vi "ini_build_objects_list.vi"(8 "error in":errorcluster, 9 "VI rel path (empty)":string, 10 "VI name (empty)":string, 11 "objects":refnum<vi>[](array[refnum])) -> (0 "error out":errorcluster, 3 "objects list":string)   [LabVIEW 2013]
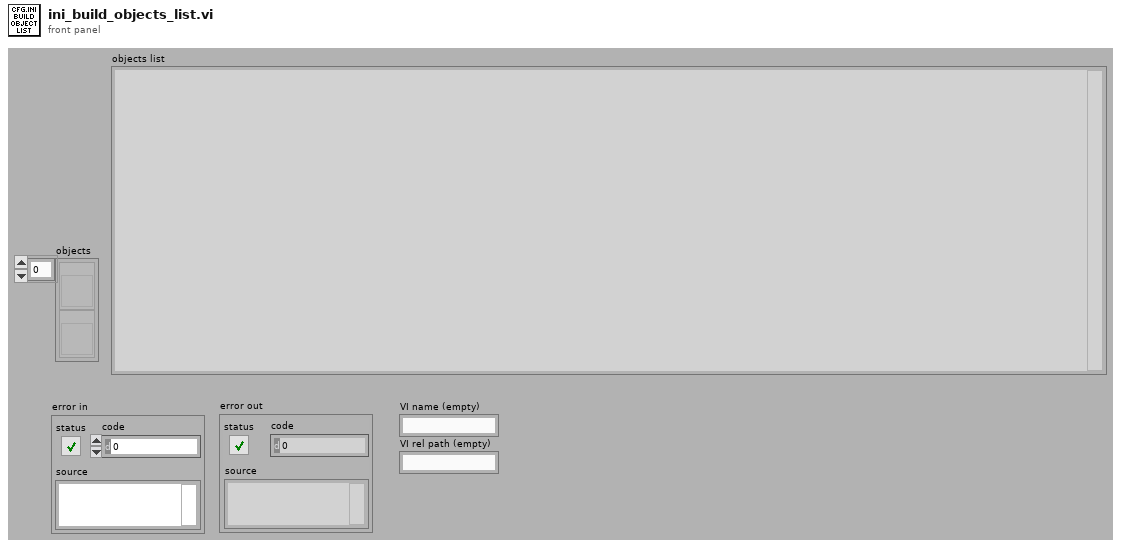
[diagram p1: front panel]
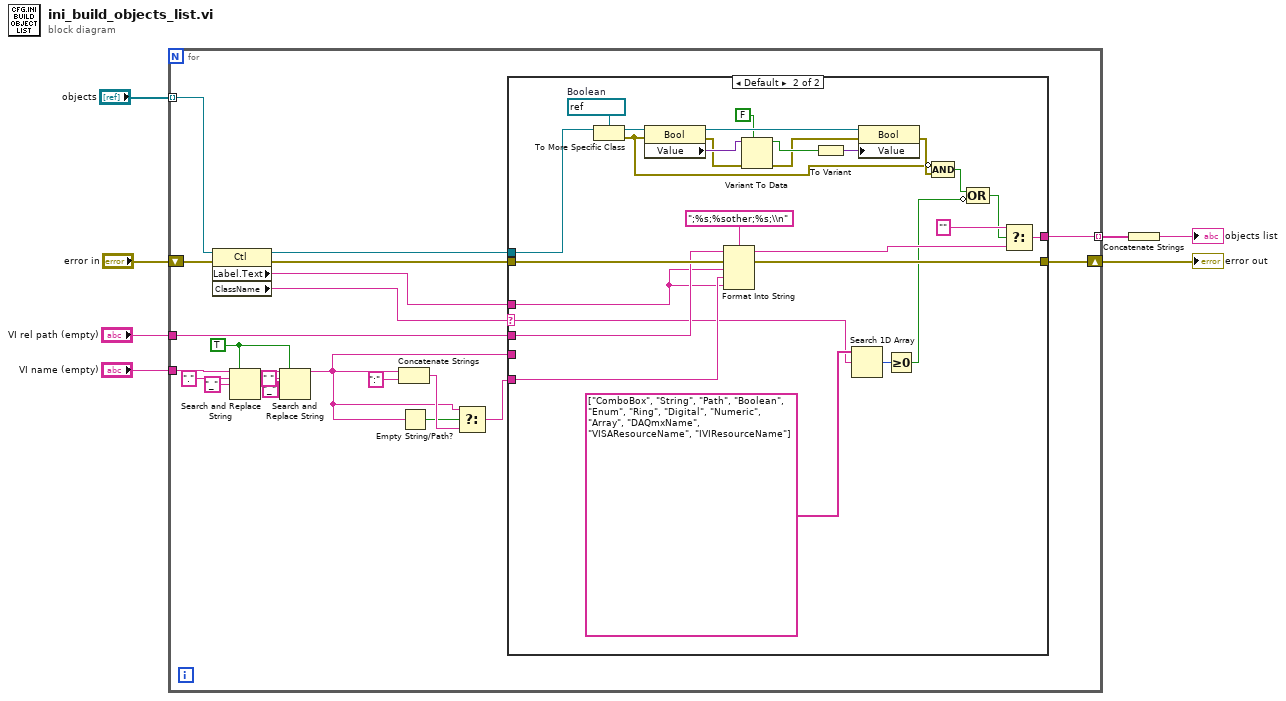
[diagram p0: block diagram]
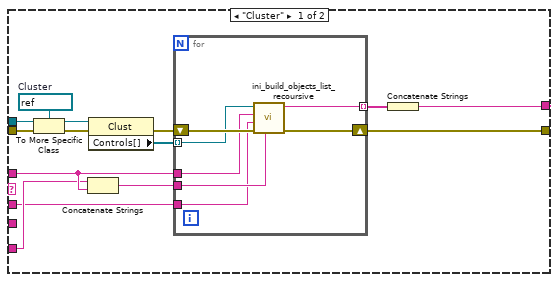
[diagram p2: hidden frame]
diagram:
  n1 = for {
    tunnel: "objects" -> [w27] mode=indexing
    shift-right: [w23] -> w5
    shift-left: "error in" -> [w28]
    tunnel: [w22] -> w4 mode=indexing
    tunnel: "VI name (empty)" -> [w16]
    tunnel: "VI rel path (empty)" -> [w13]
    w8 = TRUE ("ignore case? (F)")
    n2 = property class="Ctl"(reference=w27, error in=w28) -> (reference out=w25:refnum<vi>, error out=w24:errorcluster, "Label.Text"=w15:string, "ClassName"=w26:string)
    n3 = Search and Replace String(replace all?=w8, input string=w16, search string="." ("substring (\"\")"), replace string="_" ("replace string (\"\")")) -> (result string=w12:string)  [unwired: 4 in, 3 out]
    n4 = Search and Replace String(replace all?=w8, input string=w12, search string=" ", replace string="_" ("replace string (\"\")")) -> (result string=w11:string)  [unwired: 4 in, 3 out]
    n5 = Concatenate Strings(w11, ":" ("string")) -> (w18:string)
    n6 = Empty String/Path?(string/path=w11) -> (empty?=w14:bool)
    n7 = Select(t=w11, s=w14, f=w18) -> (s? t:f=w17:string)
    n8 = case shown="Default" w26 {
      selector: w26 -> [_ w50]
      tunnel: w25 -> [w42 w72]
      tunnel: w24 -> [w40 w75]
      tunnel: w15 -> [w31 w54]
      tunnel: [w34 w71] -> w22
      tunnel: [w33 w66] -> w23
      tunnel: w17 -> [w30 w73]
      tunnel: w13 -> [w29 w74]
      tunnel: w11 -> [_ _]
      frame "Cluster" {
        w41 = refnum<vi> refnum  # Cluster
        n9 = To More Specific Class(target class=w41, reference=w42, error in=w40) -> (specific class reference=w38:refnum<vi>, error out=w39:errorcluster)
        n10 = Concatenate Strings(w30, w31) -> (w32:string)
        n11 = property class="Clust"(reference=w38, error in=w39) -> (error out=w36:errorcluster, "Controls[]"=w37:refnum<vi>[])  [unwired: 1 out]
        n12 = for {
          tunnel: w37 -> [w48] mode=indexing
          shift-right: [w47] -> w33
          shift-left: w36 -> [w49]
          tunnel: [w46] -> w35 mode=indexing
          tunnel: w31 -> [w45]
          tunnel: w32 -> [w44]
          tunnel: w29 -> [w43]
          n13 = call "ini_build_objects_list_recoursive.vi"("base cluster"=w44, "error in"=w49, "owning vi rel path"=w43, "owner chain (empty)"=w45, "Ctl Refnum"=w48) -> ("error out"=w47:errorcluster, "item"=w46:string)  [unwired: 5 in]
        }
        n14 = Concatenate Strings(w35) -> (w34:string)
      }
      frame Default {
        w67 = refnum<vi> refnum  # Boolean
        n15 = To More Specific Class(target class=w67, reference=w72) -> (specific class reference=w68:refnum<vi>, error out=w61:errorcluster)  [unwired: 1 in]
        n16 = property class="Bool"(reference=w68, error in=w61) -> (reference out=w65:refnum<vi>, error out=w57:errorcluster, "Value"=w63:variant)
        n17 = Format Into String(format string=";%s;%sother;%s;\\n", initial string=w74, error in=w75, w54, w73, w54) -> (resulting string=w70:string, error out=w66:errorcluster)
        n18 = Variant To Data(error in=w57, type=FALSE, Variant=w63) -> (data=w62:bool, error out=w60:errorcluster)
        n19 = To Variant(anything=w62) -> (Variant=w58:variant)
        n20 = Search 1D Array(1D array=string[] ["ComboBox", "String", "Path", "Boolean", "Enum", "Ring", "Digital", "Numeric", "Array", "DAQmxName", "VISAResourceName", "IVIResourceName"], element=w50) -> (index of element=w55:i32)  [unwired: 1 in]
        n21 = property class="Bool"(reference=w65, error in=w60, "Value"=w58) -> (error out=w64:errorcluster)  [unwired: 1 out]
        n22 = Greater Or Equal To 0?(x=w55) -> (x >= 0?=w51:bool)
        n23 = Compound Arithmetic op=AND(invert w61, w64) -> (w53:bool)
        n24 = Compound Arithmetic op=OR(w53, invert w51) -> (w52:bool)
        n25 = Select(t="", s=w52, f=w70) -> (s? t:f=w71:string)
      }
    }
  }
  "error out" <- w5
  n26 = Concatenate Strings(w4) -> (→"objects list":string)
